vi "daq_muxed_thermistors.vi"(1 "index":fxp<+,3,3>, 2 "Timeout":i32) -> (0 "Timed Out?":bool)   [LabVIEW 2018]
uses:
  indexed_analog.ctl
  <vilib>/rvi/eio/common/nirviEmuTemplateMethod_errors.vi
  <vilib>/rvi/DataTransferAndStorage/Container/Common/niFpgaContainerExecOnDevCompGetState.vi
  <vilib>/rvi/Emulation/niFpgaEmulationIsFPGAContextNoSignature.vi
  <vilib>/rvi/Emulation/niFpgaSctlEmulationGetInTimedLoop.vi
  <vilib>/rvi/errors/niFpgaSetErrorForExecOnDevCompSimple.vi
  <vilib>/rvi/eio/common/nirviEmuReportErrorAndStop.vi
  <vilib>/rvi/DataTransferAndStorage/Container/Common/niFpgaContainerGetUniqueNameForEmu.vi
  <vilib>/rvi/FIFO/Fifo_Resource/nirvififoEmulationSetSize.vi
  <vilib>/rvi/FIFO/Fifo_Resource/nirviFifoEmulationQueueMgr.vi
  <instcachedir>/0/nirviFifoEmulationQueueMgr_E5CAEC123FF24DC58D834DCA3CDAA9B5.lvgen/nirviFifoEmulationQueueMgr_E5CAEC123FF24DC58D834DCA3CDAA9B5_003.vi
  <vilib>/rvi/FIFO/Fifo_Resource/nirvififoEmulationDetermineInputValidOut.vi
  <vilib>/rvi/FIFO/Fifo_Resource/nirvififoEmulationCreateLock.vi
  <vilib>/rvi/Emulation/niFpgaProcessEmulError.vi
  <vilib>/rvi/FIFO/Fifo_Resource/nirvififoEmulationObtainLock.vi
  <vilib>/rvi/FIFO/Fifo_Resource/nirvififoEmulationReleaseLock.vi
  <vilib>/rvi/occurrence/nirviWaitOnOccurrenceBase.vi
  <vilib>/rvi/errors/nirviReportUnexpectedCaseInternalError.vi
  <vilib>/rvi/errors/nirviReportUnexpectedCaseInternalError (U32).vi
  <vilib>/Utility/error.llb/Clear Errors.vi
  <vilib>/rvi/interface/RandomDataEmulation/niFpgaRandomDataHandleErrors.vi
  <vilib>/eio/EIONode/EIONode.xnode
  <vilib>/rvi/DataTransferAndStorage/Container/XNode/niFpgaContainer.xnode
  <vilib>/rvi/FIFO/Fifo_Resource/niFpgaFifoEmulationRefIn.vi
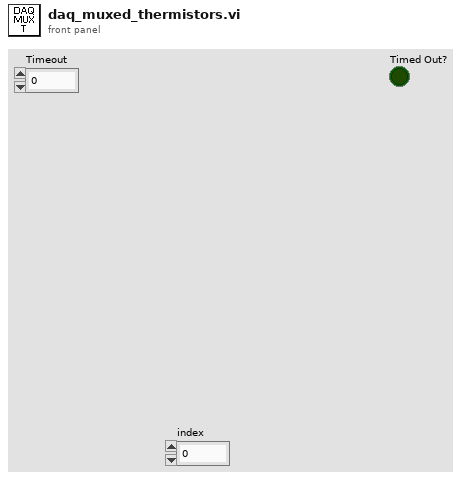
[diagram p1: front panel]
types:
  T1 = typedef "indexed_analog.ctl" = cluster{"Analog":fxp<+/-,24,5>, "Index":fxp<+,3,3>}
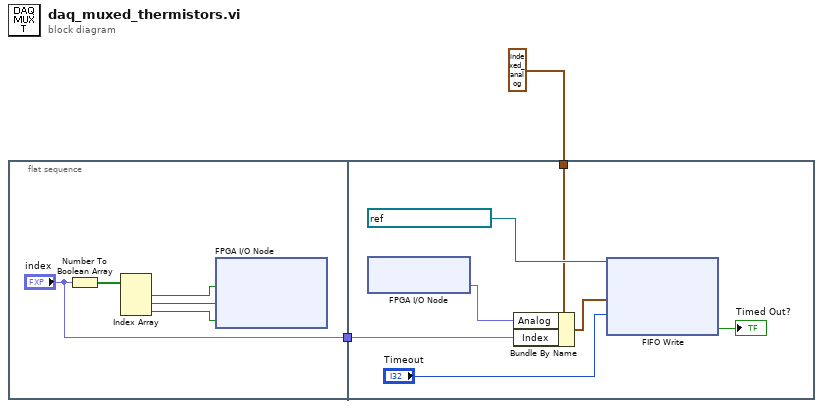
[diagram p0: block diagram]
diagram:
  n1 = flat-sequence {
    tunnel: ["index"] -> w2
    tunnel: w2 -> [w13]
    tunnel: T1 {"Analog"=0.0, "Index"=0.0} ("indexed_analog") -> [w12]
    frame #0 {
      n2 = Number To Boolean Array(number="index") -> (Boolean array=w7:bool[])
      n3 = Index Array(array=w7) -> (element #1=w6:bool, element #2=w5:bool, element #3=w4:bool)  [unwired: 3 in]
      n4 = xnode "FPGA I/O Node"("Mod2/DIO23"=w6, "Mod2/DIO24"=w5, "Mod2/DIO25"=w4) -> ()  [unwired: 3 in, 3 out]
    }
    frame #1 {
      n5 = xnode "FPGA I/O Node"() -> ("Mod1/AI11"=w8:fxp<+/-,24,5>)  [unwired: 1 in, 1 out]
      n6 = Bundle By Name(cluster=w12, "Analog"=w8, "Index"=w13) -> (w11:T1)
      n7 = xnode "FIFO Write"("Element"=w11, "Timeout"="Timeout", "FIFO In"=refnum<k21> "T_pistons_indexed") -> ("Timed Out?"=→"Timed Out?":bool)  [unwired: 1 out]
    }
  }
